vi "subGenerateDGMLContainsString.vi"(9 "Contained":set{string}(c389), 11 "Source":string) -> (1 "Links":T1)   [LabVIEW 2020, in "DefaultExtensions.lvlib" / "CGrapherDGML.lvclass"]
uses:
  CGrapherDGML.lvclass
  obj/Addons/LabVIEWItem.lvlibp/LabVIEWItem/CLabVIEWItem/ConnectionSet.ctl
  obj/Addons/LabVIEWItem.lvlibp/LabVIEWItem/CLabVIEWItem/CLabVIEWItem.lvclass
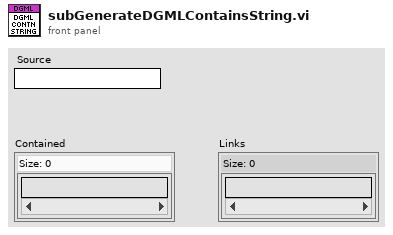
[diagram p1: front panel]
types:
  T1 = typedef "LabVIEWItem.lvlibp/CLabVIEWItem.lvclass/ConnectionSet.ctl" = set{string}
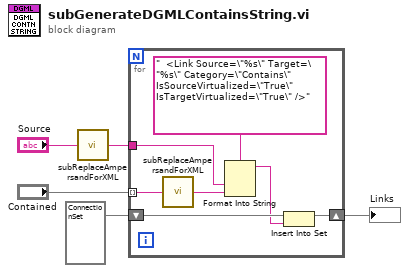
[diagram p0: block diagram]
diagram:
  n1 = call "subReplaceAmpersandForXML.vi"("String"="Source") -> ("result string"=w5:string)
  n2 = for {
    tunnel: "Contained" -> [w7] mode=indexing
    tunnel: w5 -> [w12]
    shift-right: [w9] -> w1
    shift-left: T1 {} ("set in") -> [w10]
    n3 = call "subReplaceAmpersandForXML.vi"("String"=w7) -> ("result string"=w6:string)
    n4 = Format Into String(format string="  <Link Source=\"%s\" Target=\"%s\" Category=\"Contains\" IsSourceVirtualized=\"True\" IsTargetVirtualized=\"True\" />", w12, w6) -> (resulting string=w8:string)  [unwired: 2 in, 1 out]
    n5 = Insert Into Set(10:w8, 11:w10) -> (3:w9:T1)  [unwired: 1 out]
  }
  "Links" <- w1
